vi "Main.vi"() -> ()   [LabVIEW 2014]
uses:
  experimental data.ctl
  <vilib>/Utility/sysdir.llb/System Directory Type.ctl
  <vilib>/Utility/error.llb/DialogType.ctl
  <vilib>/DAQmx/create/channels.llb/DAQmx Create Channel (AI-Voltage-Basic).vi
  <vilib>/DAQmx/create/channels.llb/DAQmx Create Channel (AO-Voltage-Basic).vi
  <vilib>/DAQmx/configure/timing.llb/DAQmx Timing (Sample Clock).vi
  <vilib>/DAQmx/write.llb/DAQmx Write (Analog DBL 1Chan 1Samp).vi
  <vilib>/Utility/config.llb/NI_LVConfig.lvlib
panel:
  out "Progress":string
  in  "Send email":bool
  in  "Email recipient":string
  in  "Number of loops to average":u16=8 min=1 step=1
  in  "Scan comments":string="These comments are saved on the screenshot image, and get emailed to you, but are NOT saved to the text data file. You have been warned."
  out "Last scan saved as":path=path "C:/Users/rajv202/Downloads/MOKE Data/2014-12-04/164027.dat"
  out "A-B Graph":cluster{dbl[], dbl[]}(graph)={[-0.07477034821619312, -0.04425183874019593, -0.013733329264198737, 0.016479995117038484, 0.04699850459303567, 0.07751701406903287, 0.10788293099765008, 0.13840144047364727, 0.16876735740226448, 0.19928586687826166, 0.22965178380687887, 0.26001770073549607, 0.2903836176641133, 0.32090212714011046, 0.3511154515213477, 0.3814813684499649, 0.4118472853785821, 0.4422132023071993, 0.47242652668843654, 0.5027924436170538, 0.5330057679982909, 0.5632190923795282, 0.5934324167607654, 0.6234931485946227, 0.6537064729758598, 0.6837672048097171, 0.7138279366435744, 0.7438886684774315, 0.7739494003112888, 0.804010132145146, 0.8339182714316232, 0.8638264107181005, 0.8937345500045778, 0.923490096743675, 0.9533982360301523, 0.9831537827692496, 1.012756736960967, 1.042512283700064, 1.0721152378917813, 1.1017181920834986, 1.131321146275216, 1.1607715079195533, 1.1902218695638904, 1.2195196386608478, 1.2489700003051851, 1.2782677694021425, 1.3074129459517196, 1.336710715048677, 1.3657032990508744, 1.3948484756004518, 1.423841059602649, 1.4528336436048463, 1.4816736350596638, 1.510513626514481, 1.5393536179692984, 1.5680410168767358, 1.596575823236793, 1.6252632221442305, 1.653645435956908, 1.6821802423169652, 1.7105624561296426, 1.7387920773949401, 1.7670216986602374, 1.7952513199255349, 1.8233283486434522, 1.8512527848139897, 1.8791772209845272, 1.9071016571550645, 1.934873500778222, 1.9624927518539994, 1.990112002929777, 2.0177312540055543, 2.045197912533952, 2.0725119785149695, 2.0998260444959866, 2.1269875179296243, 2.154148991363262, 2.1811578722495195, 2.2080141605883967, 2.2348704489272744, 2.261574144718772, 2.2882778405102693, 2.314828943754387, 2.3413800469985047, 2.3676259651478624, 2.3940244758445997, 2.4201178014465774, 2.446211127048555, 2.4721518601031525, 2.4980925931577502, 2.523880733664968, 2.5495162816248054, 2.575151829584643, 2.6006347849971005, 2.6259651478621784, 2.6511429181798762, 2.6763206884975737, 2.7013458662678915, 2.726371044038209, 2.751091036713767, 2.775811029389325, 2.8005310220648822, 2.82494582964568, 2.8493606372264777, 2.8736228522598957, 2.897732474745933, 2.921689504684591, 2.945646534623249, 2.969450972014527, 2.993102816858425, 3.0166020691549424, 3.0401013214514605, 3.063295388653218, 3.0864894558549762, 3.109530930509354, 3.1324198126163516, 3.1553086947233497, 3.1778923917355875, 3.2004760887478256, 3.2229071932126834, 3.2451857051301616, 3.2673116245002594, 3.2892849513229776, 3.3112582781456954, 3.3329264198736532, 3.3545945616016115, 3.3761101107821894, 3.3974730674153872, 3.4186834315012056, 3.4397412030396435, 3.4606463820307014, 3.48139896847438, 3.5019989623706778, 3.5225989562669757, 3.542893765068514, 3.563188573870052, 3.58317819757683, 3.6031678212836087, 3.6230048524430067, 3.642536698507645, 3.662068544572283, 3.6814477980895415, 3.7006744590594196, 3.7197485274819178, 3.738670003357036, 3.757438886684774, 3.7759025849177528, 3.794366283150731, 3.8126773888363292, 3.8308359019745475, 3.8488418225653858, 3.866695150608844, 3.884395886104923, 3.901944029053621, 3.9191869869075595, 3.936429944761498, 3.9535203100680563, 3.9704580828272347, 3.987090670491653, 4.0037232581560716, 4.0200506607257305, 4.0363780632953885, 4.0524002807702875, 4.0684224982451855, 4.0841395306253245, 4.099703970458083, 4.115115817743462, 4.13037507248146, 4.145481734672079, 4.160435804315317, 4.175237281411176, 4.1897335734122745, 4.204229865413374, 4.218420972319712, 4.23261207922605, 4.246498001037629], [0.7960753196813868, 0.8261360515152439, 0.8560441908017212, 0.8859523300881985, 0.9158604693746757, 0.945768608661153, 0.9755241554002503, 1.0052797021393476, 1.0350352488784447, 1.064790795617542, 1.0943937498092593, 1.1239967040009766, 1.153447065645314, 1.183050019837031, 1.2125003814813684, 1.2417981505783258, 1.271248512222663, 1.3005462813196202, 1.3298440504165776, 1.358989226966155, 1.3881344035157324, 1.4171269875179295, 1.446272164067507, 1.4751121555223243, 1.5041047395245217, 1.532944730979339, 1.5616321298867764, 1.5904721213415938, 1.619006927701651, 1.6476943266090884, 1.6762291329691459, 1.7046113467818231, 1.7329935605945006, 1.7613757744071779, 1.7896053956724753, 1.8176824243903928, 1.8459120456556901, 1.8738364818262276, 1.901760917996765, 1.9296853541673025, 1.95745719779046, 1.9852290414136173, 2.012848292489395, 2.0403149510177925, 2.0677816095461896, 2.095248268074587, 2.122562334055605, 2.1497238074892424, 2.1768852809228796, 2.203894161809137, 2.230903042695395, 2.257759331034272, 2.2844630268257697, 2.3111667226172674, 2.337717825861385, 2.3642689291055023, 2.39066743980224, 2.416913357951598, 2.443159276100955, 2.469252601702933, 2.4951933347575306, 2.521134067812128, 2.5469222083193457, 2.5727103488265635, 2.598193304239021, 2.6236762596514787, 2.6491592150639365, 2.674489577929014, 2.6996673482467117, 2.724692526017029, 2.749565111239967, 2.774437696462905, 2.7991576891384624, 2.8238776818140203, 2.848292489394818, 2.8727072969756158, 2.8969695120090333, 2.9212317270424513, 2.945188756981109, 2.969145786919767, 2.992950224311045, 3.0166020691549424, 3.0402539139988405, 3.063600573747978, 3.086947233497116, 3.110141300698874, 3.133182775353252, 3.1562242500076296, 3.1789605395672473, 3.2016968291268655, 3.224280526139103, 3.2467116306039614, 3.268990142521439, 3.2912686544389174, 3.313241981261635, 3.335215308084353, 3.3568834498123112, 3.378551591540269, 3.4000671407208474, 3.4214300973540452, 3.442793053987243, 3.4638508255256815, 3.4847560045167394, 3.5056611835077973, 3.5262611774040957, 3.5468611713003937, 3.5671559801019317, 3.58745078890347, 3.607593005157628, 3.627582628864406, 3.6474196600238042, 3.6671040986358228, 3.686635944700461, 3.706015198217719, 3.725241859187597, 3.7443159276100957, 3.763237403485214, 3.782006286812952, 3.8006225775933102, 3.8190862758262885, 3.837397381511887, 3.8557084871974854, 3.8737144077883237, 3.891567735831782, 3.9092684713278603, 3.9268166142765586, 3.944212164677877, 3.9614551225318158, 3.978545487838374, 3.9954832605975525, 4.0122684408093505, 4.028901028473769, 4.045228431043427, 4.061555833613086, 4.077730643635364, 4.093600268562883, 4.1094698934904015, 4.1250343333231605, 4.140598773155919, 4.155858027893918, 4.170964690084536, 4.185918759727775, 4.200720236823633, 4.215369121372112, 4.2298654133732105, 4.24420911282693, 4.258247627185888, 4.272286141544847, 4.2860194708090456, 4.299600207525865, 4.313028351695303, 4.326303903317362, 4.339426862392041, 4.352397228919339, 4.365062410351879, 4.377727591784417, 4.390087588122196, 4.402294991912595, 4.414349803155614, 4.426252021851253, 4.438001647999512, 4.44944608905301, 4.46089053010651, 4.4720297860652485, 4.483016449476607, 4.493850520340587, 4.5043794061098055, 4.514908291879024, 4.525131992553484, 4.535203100680563, 4.5451216162602615, 4.554887539292581, 4.56450086977752, 4.573809015167699, 4.582964568010499, 4.591967528305918]}
  out "A+B Graph":cluster{dbl[], dbl[]}(graph)={[-0.07477034821619312, -0.04425183874019593, -0.013733329264198737, 0.016479995117038484, 0.04699850459303567, 0.07751701406903287, 0.10788293099765008, 0.13840144047364727, 0.16876735740226448, 0.19928586687826166, 0.22965178380687887, 0.26001770073549607, 0.2903836176641133, 0.32090212714011046, 0.3511154515213477, 0.3814813684499649, 0.4118472853785821, 0.4422132023071993, 0.47242652668843654, 0.5027924436170538, 0.5330057679982909, 0.5632190923795282, 0.5934324167607654, 0.6234931485946227, 0.6537064729758598, 0.6837672048097171, 0.7138279366435744, 0.7438886684774315, 0.7739494003112888, 0.804010132145146, 0.8339182714316232, 0.8638264107181005, 0.8937345500045778, 0.923490096743675, 0.9533982360301523, 0.9831537827692496, 1.012756736960967, 1.042512283700064, 1.0721152378917813, 1.1017181920834986, 1.131321146275216, 1.1607715079195533, 1.1902218695638904, 1.2195196386608478, 1.2489700003051851, 1.2782677694021425, 1.3074129459517196, 1.336710715048677, 1.3657032990508744, 1.3948484756004518, 1.423841059602649, 1.4528336436048463, 1.4816736350596638, 1.510513626514481, 1.5393536179692984, 1.5680410168767358, 1.596575823236793, 1.6252632221442305, 1.653645435956908, 1.6821802423169652, 1.7105624561296426, 1.7387920773949401, 1.7670216986602374, 1.7952513199255349, 1.8233283486434522, 1.8512527848139897, 1.8791772209845272, 1.9071016571550645, 1.934873500778222, 1.9624927518539994, 1.990112002929777, 2.0177312540055543, 2.045197912533952, 2.0725119785149695, 2.0998260444959866, 2.1269875179296243, 2.154148991363262, 2.1811578722495195, 2.2080141605883967, 2.2348704489272744, 2.261574144718772, 2.2882778405102693, 2.314828943754387, 2.3413800469985047, 2.3676259651478624, 2.3940244758445997, 2.4201178014465774, 2.446211127048555, 2.4721518601031525, 2.4980925931577502, 2.523880733664968, 2.5495162816248054, 2.575151829584643, 2.6006347849971005, 2.6259651478621784, 2.6511429181798762, 2.6763206884975737, 2.7013458662678915, 2.726371044038209, 2.751091036713767, 2.775811029389325, 2.8005310220648822, 2.82494582964568, 2.8493606372264777, 2.8736228522598957, 2.897732474745933, 2.921689504684591, 2.945646534623249, 2.969450972014527, 2.993102816858425, 3.0166020691549424, 3.0401013214514605, 3.063295388653218, 3.0864894558549762, 3.109530930509354, 3.1324198126163516, 3.1553086947233497, 3.1778923917355875, 3.2004760887478256, 3.2229071932126834, 3.2451857051301616, 3.2673116245002594, 3.2892849513229776, 3.3112582781456954, 3.3329264198736532, 3.3545945616016115, 3.3761101107821894, 3.3974730674153872, 3.4186834315012056, 3.4397412030396435, 3.4606463820307014, 3.48139896847438, 3.5019989623706778, 3.5225989562669757, 3.542893765068514, 3.563188573870052, 3.58317819757683, 3.6031678212836087, 3.6230048524430067, 3.642536698507645, 3.662068544572283, 3.6814477980895415, 3.7006744590594196, 3.7197485274819178, 3.738670003357036, 3.757438886684774, 3.7759025849177528, 3.794366283150731, 3.8126773888363292, 3.8308359019745475, 3.8488418225653858, 3.866695150608844, 3.884395886104923, 3.901944029053621, 3.9191869869075595, 3.936429944761498, 3.9535203100680563, 3.9704580828272347, 3.987090670491653, 4.0037232581560716, 4.0200506607257305, 4.0363780632953885, 4.0524002807702875, 4.0684224982451855, 4.0841395306253245, 4.099703970458083, 4.115115817743462, 4.13037507248146, 4.145481734672079, 4.160435804315317, 4.175237281411176, 4.1897335734122745, 4.204229865413374, 4.218420972319712, 4.23261207922605, 4.246498001037629], [0.43214209418012023, 0.46250801110873746, 0.49287392803735464, 0.5230872524185919, 0.5534531693472091, 0.5836664937284463, 0.6140324106570635, 0.6442457350383007, 0.674459059419538, 0.7045197912533951, 0.7347331156346324, 0.7647938474684897, 0.7948545793023468, 0.8249153111362041, 0.8549760429700614, 0.8850367748039186, 0.9149449140903958, 0.9448530533768731, 0.9747611926633504, 1.0045167394024477, 1.0344248786889247, 1.064180425428022, 1.0939359721671194, 1.1235389263588367, 1.153141880550554, 1.182744834742271, 1.2123477889339884, 1.2417981505783258, 1.271248512222663, 1.3006988738670002, 1.3299966429639576, 1.359294412060915, 1.3885921811578723, 1.4177373577074495, 1.4468825342570268, 1.4760277108066042, 1.5050202948088016, 1.5338602862636188, 1.5628528702658162, 1.5916928617206336, 1.6203802606280708, 1.6492202520828882, 1.6777550584429457, 1.706442457350383, 1.7348246711630604, 1.7633594775231178, 1.791741691335795, 1.8199713126010926, 1.84820093386639, 1.8764305551316873, 1.9045075838496048, 1.9325846125675221, 1.9605090487380596, 1.988280892361217, 2.0160527359843745, 2.043824579607532, 2.0714438306833096, 2.0989104892117068, 2.1263771477401043, 2.153843806268502, 2.1811578722495195, 2.2083193456831567, 2.2354808191167943, 2.262489700003052, 2.2893459883419296, 2.316202276680807, 2.3430585650196845, 2.369609668263802, 2.3963133640552994, 2.422711874752037, 2.449110385448775, 2.475356303598132, 2.50160222174749, 2.5276955473494676, 2.553636280404065, 2.5795770134586626, 2.6053651539658804, 2.6310007019257178, 2.6566362498855556, 2.6821192052980134, 2.707449568163091, 2.7327799310281686, 2.7579577013458665, 2.782982879116184, 2.807855464339122, 2.8327280495620593, 2.857448042237617, 2.8820154423657947, 2.9065828424939726, 2.9309976500747705, 2.955259865108188, 2.979369487594226, 3.0034791100802636, 3.0272835474715416, 3.051087984862819, 3.074739829706717, 3.098391674550615, 3.121738334299753, 3.1450849940488905, 3.1682790612506486, 3.1913205359050263, 3.2142094180120244, 3.237098300119022, 3.2598345896786403, 3.282265694143498, 3.3046967986083557, 3.326975310525834, 3.3492538224433117, 3.37122714926603, 3.3932004760887478, 3.414868617816706, 3.436536759544664, 3.4580523087252417, 3.47941526535844, 3.500625629444258, 3.521683400982696, 3.542588579973754, 3.563493758964812, 3.58409375286111, 3.6046937467574085, 3.6249885555589465, 3.6452833643604845, 3.665425580614643, 3.685262611774041, 3.705099642933439, 3.724784081545457, 3.7443159276100957, 3.763695181127354, 3.782921842097232, 3.80199591051973, 3.8209173863948487, 3.839686269722587, 3.858302560502945, 3.8767662587359233, 3.8950773644215215, 3.91323587755974, 3.9312417981505785, 3.949095126194037, 3.966795861690115, 3.9843440046388134, 4.001739555040132, 4.018829920346691, 4.035920285653249, 4.052858058412427, 4.069643238624225, 4.086275826288644, 4.102603228858302, 4.118930631427961, 4.134952848902859, 4.150975066377758, 4.166692098757896, 4.182409131138035, 4.1978209784234135, 4.213080233161413, 4.228186895352031, 4.24314096499527, 4.257942442091128, 4.272591326639607, 4.286935026093325, 4.301278725547045, 4.315317239906003, 4.329355754264962, 4.3430890835291605, 4.356669820245979, 4.370097964415418, 4.3833735160374765, 4.396496475112156, 4.409314249092074, 4.422132023071994, 4.434644611957152, 4.447004608294931, 4.45921201208533, 4.471266823328349, 4.483169042023987, 4.494766075624867, 4.506363109225745]}
  out "Estimated finish time":timestamp=timestamp(3500556027.964023 s since 1904-01-01) format="%<%I:%M %p>T"
  out "Progress Bar":u8(slide)=100 scale=0.0..100.0
  in  "Stop Button":bool
  in  "Magnet Ramp Segments":string[][](table)=[["0", "-1", "8"], ["-1", "1", "80"], ["1", "-1", "80"], ["-1", "0", "8"]]
  in  "Field Settle Time (msec)":dbl=400.0
  in  "Output Voltage Limit +/-":dbl=5.0 min=0.0 max=10.0 step=0.0001 format="%.2f"
  in  "Input Voltage Limit +/-":dbl=5.0 min=0.0 max=10.0 step=0.0001 format="%.2f"
  in  "Magnet Power Supply Channel":tag="Dev1/ao0"
  in  "A-B Channel":tag="Dev1/ai1"
  in  "A+B Channel":tag="Dev1/ai0"
  in  "Hall Probe Channel":tag="Dev1/ai2"
  in  "Start Button":bool
  # "Generic Small MOKE"
  # "Released 2015-01-16 16:23"
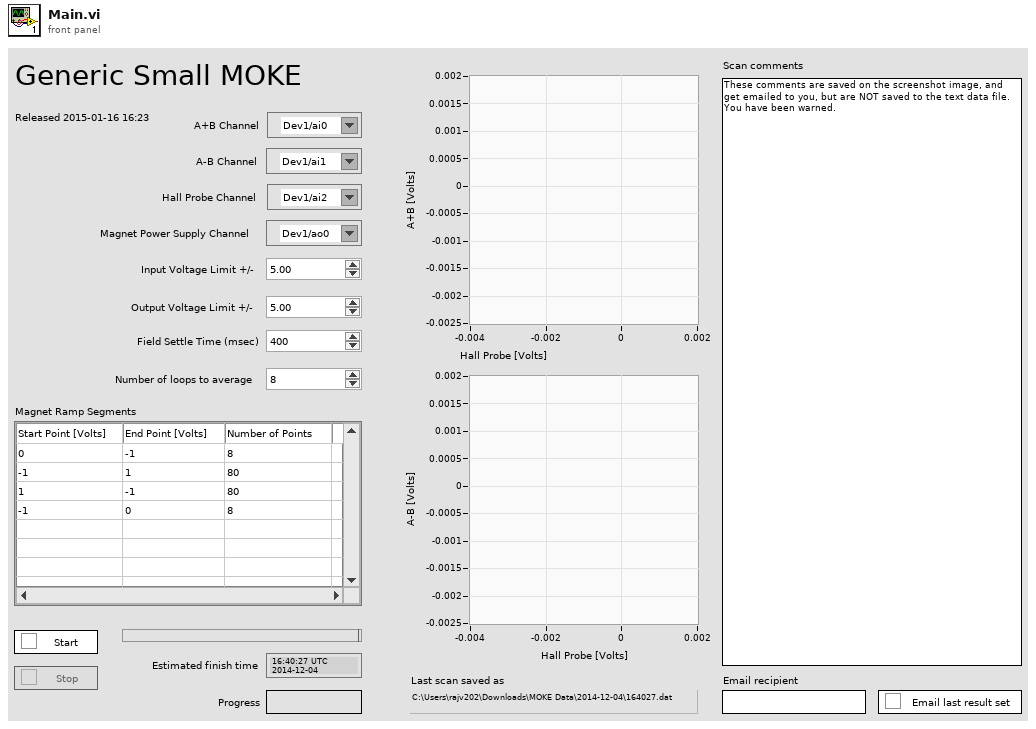
[diagram p1: front panel]
types:
  T1 = typedef "System Directory Type.ctl" = i32
  T2 = typedef "experimental data.ctl" = cluster{"Hall Probe":dbl, "A+B":dbl, "A-B":dbl, "Progress":u32[]}
  T3 = typedef "NI_LVConfig.lvlib/Config Data RefNum.ctl" = refnum<k1>
  T4 = enum8{"Enabled", "Disabled", "Disabled and Grayed Out"}
  T5 = enum16{"open", "replace", "create", "open or create", "replace or create", "replace or create with confirmation"}
  T6 = typedef "imagedata.ctl" = cluster{"image type":i32, "image depth":i32, "image":u8[], "mask":u8[], "colors":u32[], "Rectangle":cluster{"left":i16, "top":i16, "right":i16, "bottom":i16}}
  T7 = typedef "DialogType.ctl" = u16
  T8 = cluster{"New data array":dbl[], "New data array":dbl[]}
  T9 = cluster{"Server address":string, "Use TLS?":bool, "Username":string, "Password":string, "Recipient":string}
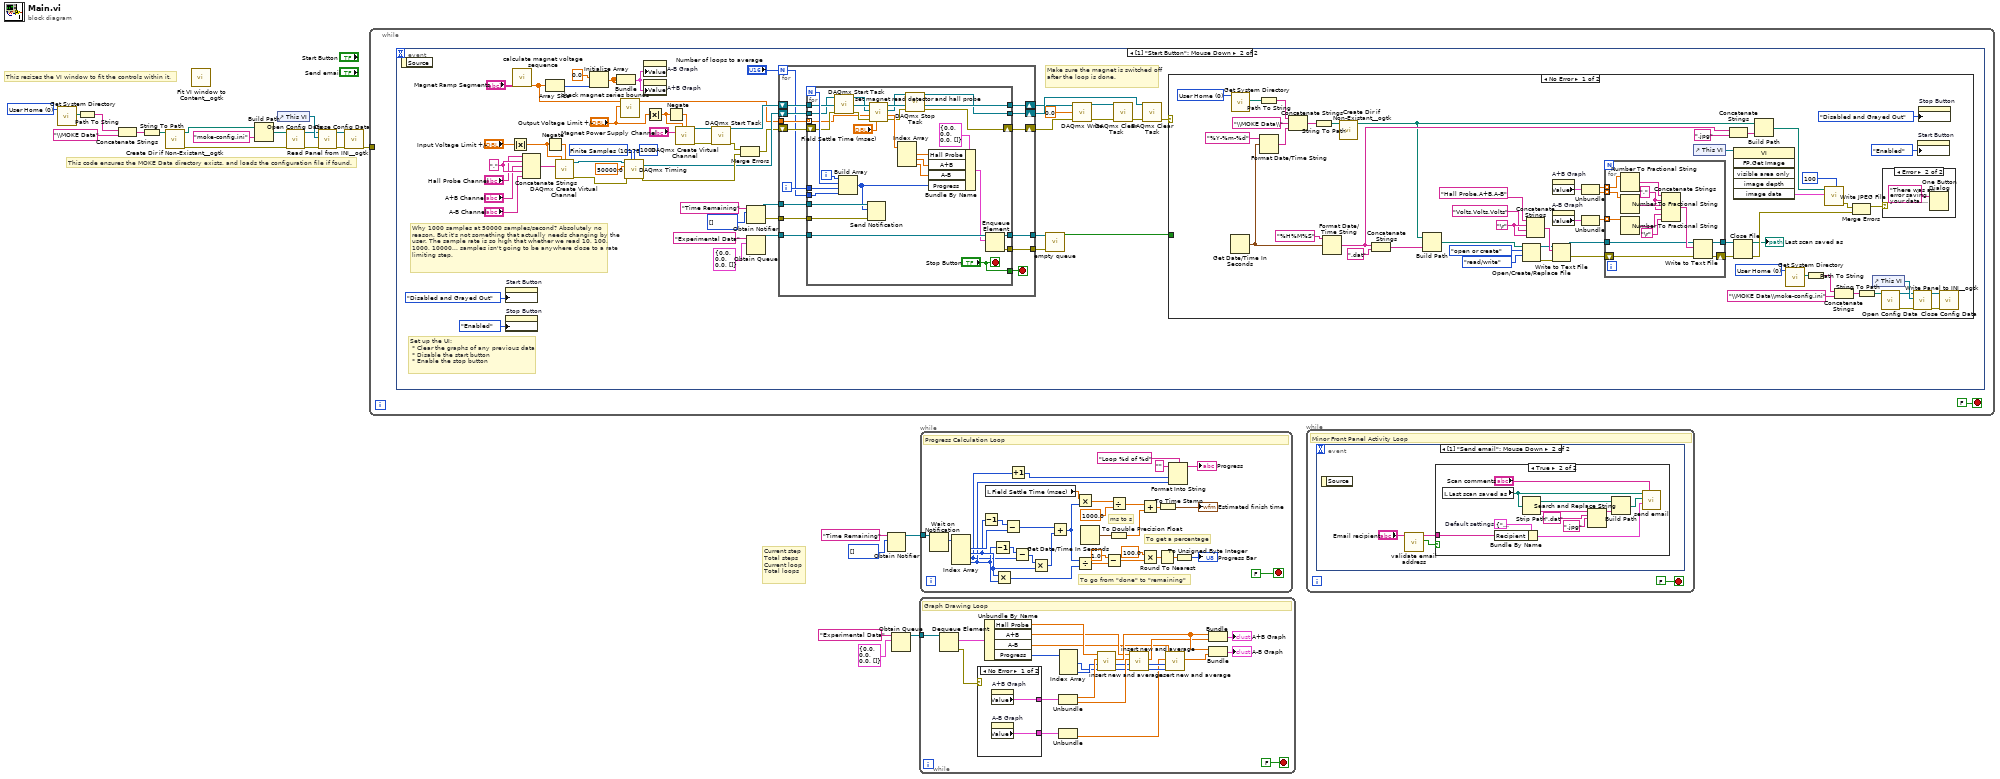
[diagram p0: block diagram]
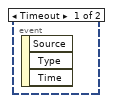
[diagram p2: hidden frame]
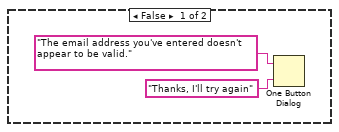
[diagram p3: hidden frame]
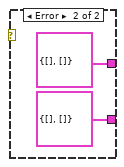
[diagram p4: hidden frame]
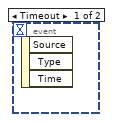
[diagram p5: hidden frame]
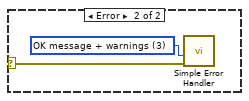
[diagram p7: hidden frame]
diagram:
  w16 = T1 0 items=["User Home"=0, "User Desktop"=1, "User Documents"=2, "User Application Data"=3, "User Preferences"=4, "User Temporary"=5, "Public Documents"=6, "Public Application Data"=7, "Public Preferences"=8, "Public Cache"=13, "System Core Libraries"=9, "System Installed Libraries"=10, "Application Files"=11, "Boot Volume Root"=12] ("system directory type")
  # "This code ensures the MOKE Data directory exists, and loads the configuration file if found."
  # "This resizes the VI window to fit the controls within it."
  # "Current step\nTotal steps\nCurrent loop\nTotal loops"
  n1 = call <vilib>:"Get System Directory.vi"("system directory type"=w16) -> ("system directory"=w15:path)  [unwired: 10 in]
  n2 = Path To String(path=w15) -> (string=w14:string)
  n3 = Concatenate Strings(w14, "\\MOKE Data" ("string")) -> (w13:string)
  n4 = String To Path(string=w13) -> (path=w5:path)
  n5 = call <userlib>:"Create Dir if Non-Existant__ogtk.vi"("Directory Path"=w5) -> ("error out"=w4:errorcluster, "dup Directory Path"=w2:path)  [unwired: 8 in, 1 out]
  n6 = call <userlib>:"Fit VI window to Content__ogtk.vi"() -> ()  [unwired: 6 in, 2 out]
  n7 = Build Path(base path=w2, name or relative path="moke-config.ini") -> (appended path=w3:path)
  n8 = control-ref of="This VI"() -> (w12:refnum<vi>)
  n9 = call <vilib>:"Open Config Data.vi"("error in (no error)"=w4, "configuration file path"=w3) -> ("error out"=w10:errorcluster, "refnum"=w11:T3)  [unwired: 7 in, 1 out]
  n10 = call <userlib>:"Read Panel from INI__ogtk.vi"("error in (no error)"=w10, "VI ref"=w12, "refnum"=w11) -> ("error out"=w8:errorcluster, "refnum out"=w9:T3)  [unwired: 7 in]
  n11 = call <vilib>:"Close Config Data.vi"("error in (no error)"=w8, "refnum"=w9) -> ("error out"=w6:errorcluster)  [unwired: 8 in, 1 out]
  n12 = while {
    tunnel: w6 -> [_]
    stop <- FALSE stop-if-true
    n13 = event shown="[1] \"Start Button\": Mouse Down" {
      selector: _ -> [_ _]
      dyn-events: _ -> [_ _]
      timeout: _ -> [_ _]
      event Timeout {
        n14 = event-data() -> ()  [unwired: 1 in, 3 out]
      }
      event "Start Button": Mouse Down {
        w34 = 10178 items=["Finite Samples"=10178, "Continuous Samples"=10123, "Hardware Timed Single Point"=12522] ("sample mode")
        w75 = ","
        # "Why 1000 samples at 50000 samples/second? Absolutely no reason. But it's not something that actually needs changing by the user. The sample rate is so high that whether we read 10, 100, 1000, 10000... samples isn't going to be anywhere close to a rate limiting step."
        # "Make sure the magnet is switched off after the loop is done."
        # "Set up the UI:\n * Clear the graphs of any previous data\n * Disable the start button\n * Enable the stop button"
        n15 = event-data() -> ()  [unwired: 1 in, 1 out]
        n16 = property on="Start Button" class="Bool (strict)"("DisabledEnum"=T4."Disabled and Grayed Out" ("Disabled")) -> ()  [unwired: 2 in, 2 out]
        n17 = property on="Stop Button" class="Bool"("DisabledEnum"=T4."Enabled" ("Disabled")) -> ()  [unwired: 2 in, 2 out]
        n18 = Absolute Value(x="Input Voltage Limit +/-") -> (abs(x)=w68:dbl)
        n19 = call "calculate magnet voltage sequence.vi"("Magnet Ramp Segments"="Magnet Ramp Segments") -> ("Magnet Voltage Sequence"=w36:dbl[])  [unwired: 8 in]
        n20 = Concatenate Strings("Hall Probe Channel", w75, "A+B Channel", w75, "A-B Channel") -> (w71:string)
        n21 = Array Size(array=w36) -> (size(s)=w42:i32)
        n22 = Negate(x=w68) -> (-x=w70:dbl)
        n23 = call-poly <vilib>:"DAQmx Create Virtual Channel.vi"("maximum value"=w68, "minimum value"=w70, "physical channels"=w71) -> ("task out"=w35:refnum<k21>, "error out"=w32:errorcluster)  [unwired: 11 in]
        n24 = Initialize Array(0.0 ("element"), w42) -> (w41:dbl[])
        n25 = Bundle(w41, w41) -> (w40:cluster{dbl[], dbl[]})  [unwired: 1 in]
        n26 = call "check magnet series bounds.vi"("Output Voltage Limit"="Output Voltage Limit +/-", "Magnet Voltage Sequence"=w36) -> ("Magnet Voltage Sequence"=w27:dbl[])  [unwired: 9 in]
        n27 = call-poly <vilib>:"DAQmx Timing.vi"("task/channels in"=w35, "sample mode"=w34, "samples per channel"=1000, "rate"=50000.0, "error in"=w32) -> ("task out"=w30:refnum<k21>, "error out"=w31:errorcluster)  [unwired: 9 in]
        n28 = property on="A-B Graph" class="XYGraph (strict)"("Value"=w40) -> ()  [unwired: 2 in, 2 out]
        n29 = property on="A+B Graph" class="XYGraph (strict)"("Value"=w40) -> ()  [unwired: 2 in, 2 out]
        n30 = Absolute Value(x="Output Voltage Limit +/-") -> (abs(x)=w66:dbl)
        n31 = Negate(x=w66) -> (-x=w67:dbl)
        n32 = call-poly <vilib>:"DAQmx Create Virtual Channel.vi"("maximum value"=w66, "minimum value"=w67, "physical channels"="Magnet Power Supply Channel") -> ("task out"=w52:refnum<k21>, "error out"=w65:errorcluster)  [unwired: 11 in]
        n33 = call <vilib>:"DAQmx Start Task.vi"("task/channels in"=w52, "error in"=w65) -> ("task out"=w63:refnum<k21>, "error out"=w64:errorcluster)  [unwired: 12 in]
        n34 = Merge Errors(w64, w31) -> (w29:errorcluster)
        n35 = Obtain Notifier(name (unnamed)="Time Remaining", notification data type=i32[] []) -> (notifier out=w59:refnum<notifier>, error out=w46:errorcluster)  [unwired: 2 in, 1 out]
        n36 = Obtain Queue(name (unnamed)="Experimental Data", element data type=T2 {"Hall Probe"=0.0, "A+B"=0.0, "A-B"=0.0, "Progress"=[]}) -> (queue out=w55:refnum<queue>)  [unwired: 3 in, 2 out]
        n37 = for {
          N: "Number of loops to average" -> [w78]
          tunnel: w59 -> [w87]
          tunnel: w27 -> [w86]
          tunnel: w55 -> [w85]
          tunnel: w46 -> [w81]
          shift-right: [w84] -> w54
          shift-left: w30 -> [w90]
          shift-right: [w82] -> w48
          shift-left: w63 -> [w89]
          shift-right: [w83] -> w51
          shift-left: w29 -> [w88]
          tunnel: [w77] -> w39
          tunnel: [w76] -> w38
          i -> [w79]
          stop <- w80 stop-if-true
          n38 = for {
            N -> [w117]
            tunnel: w90 -> [w95]
            tunnel: w89 -> [w115]
            shift-right: [w99] -> w83
            shift-left: w88 -> [w93]
            tunnel: w86 -> [w91] mode=indexing
            tunnel: w87 -> [w119]
            tunnel: w85 -> [w116]
            tunnel: [w114] -> w82
            tunnel: [w96] -> w84
            tunnel: w81 -> [w112]
            tunnel: ["Stop Button"] -> w80
            tunnel: w79 -> [w108]
            tunnel: w78 -> [w107]
            tunnel: [w103] -> w77
            tunnel: [w102] -> w76
            i -> [w118]
            stop <- "Stop Button" stop-if-true
            n39 = call <vilib>:"DAQmx Start Task.vi"("task/channels in"=w95, "error in"=w93) -> ("task out"=w94:refnum<k21>, "error out"=w92:errorcluster)  [unwired: 12 in]
            n40 = Build Array(w118, w117, w108, w107) -> (w104:i32[])
            n41 = Send Notification(notification=w104, notifier=w119, error in (no error)=w112) -> ()  [unwired: 2 out]
            n42 = call "set magnet read detector and hall probe.vi"("Field settle time (400 msec)"="Field Settle Time (msec)", "error in (no error)"=w92, "Magnet voltage"=w91, "Input task"=w94, "Output task"=w115) -> ("error out"=w98:errorcluster, "Data"=w111:dbl[], "Input task"=w97:refnum<k21>, "Output task"=w114:refnum<k21>)  [unwired: 3 in]
            n43 = Index Array(array=w111) -> (element #1=w106:dbl, element #2=w100:dbl, element #3=w105:dbl)  [unwired: 3 in]
            n44 = call <vilib>:"DAQmx Stop Task.vi"("task/channels in"=w97, "error in"=w98) -> ("task out"=w96:refnum<k21>, "error out"=w99:errorcluster)  [unwired: 12 in]
            n45 = Bundle By Name(cluster=T2 {"Hall Probe"=0.0, "A+B"=0.0, "A-B"=0.0, "Progress"=[]}, "Hall Probe"=w106, "A+B"=w100, "A-B"=w105, "Progress"=w104) -> (w109:T2)
            n46 = Enqueue Element(queue=w116, element=w109) -> (queue out=w102:refnum<queue>, error out=w103:errorcluster)  [unwired: 2 in, 1 out]
          }
        }
        n47 = call "empty queue.vi"("error in (no error)"=w39, "Queue in"=w38) -> ("Queue emptied?"=w37:bool)  [unwired: 9 in]
        n48 = call-poly <vilib>:"DAQmx Write.vi"("task/channels in"=w48, "data"=0.0, "error in"=w51) -> ("task out"=w49:refnum<k21>, "error out"=w50:errorcluster)  [unwired: 10 in, 1 out]
        n49 = call <vilib>:"DAQmx Clear Task.vi"("task in"=w49, "error in"=w50) -> ("error out"=w62:errorcluster)  [unwired: 13 in]
        n50 = call <vilib>:"DAQmx Clear Task.vi"("task in"=w54, "error in"=w62) -> ("error out"=w24:errorcluster)  [unwired: 13 in]
        n51 = case shown="No Error" w24 {
          selector: w24 -> [_ w189]
          tunnel: w37 -> [_ _]
          frame No Error {
            w138 = T1 0 items=["User Home"=0, "User Desktop"=1, "User Documents"=2, "User Application Data"=3, "User Preferences"=4, "User Temporary"=5, "Public Documents"=6, "Public Application Data"=7, "Public Preferences"=8, "Public Cache"=13, "System Core Libraries"=9, "System Installed Libraries"=10, "Application Files"=11, "Boot Volume Root"=12] ("system directory type")
            w141 = T1 0 items=["User Home"=0, "User Desktop"=1, "User Documents"=2, "User Application Data"=3, "User Preferences"=4, "User Temporary"=5, "Public Documents"=6, "Public Application Data"=7, "Public Preferences"=8, "Public Cache"=13, "System Core Libraries"=9, "System Installed Libraries"=10, "Application Files"=11, "Boot Volume Root"=12] ("system directory type")
            w147 = "\r"
            n52 = Get Date/Time In Seconds() -> (seconds since 1Jan1904=w172:timestamp)
            n53 = call <vilib>:"Get System Directory.vi"("system directory type"=w141) -> ("system directory"=w140:path)  [unwired: 10 in]
            n54 = Path To String(path=w140) -> (string=w139:string)
            n55 = Format Date/Time String(time format string (%c)="%Y-%m-%d", seconds (now)=w172) -> (date/time string=w124:string)  [unwired: 1 in]
            n56 = Concatenate Strings(w139, "\\MOKE Data\\" ("string"), w124) -> (w134:string)
            n57 = String To Path(string=w134) -> (path=w173:path)
            n58 = Format Date/Time String(time format string (%c)="%H%M%S", seconds (now)=w172) -> (date/time string=w153:string)  [unwired: 1 in]
            n59 = call <userlib>:"Create Dir if Non-Existant__ogtk.vi"("Directory Path"=w173) -> ("dup Directory Path"=w151:path)  [unwired: 8 in, 2 out]
            n60 = Concatenate Strings(w153, ".dat" ("string")) -> (w170:string)
            n61 = Build Path(base path=w151, name or relative path=w170) -> (appended path=w144:path)
            n62 = Open/Create/Replace File(file path (use dialog)=w144, operation (0:open)=T5."open or create", access (0:read/write)=enum16{"read/write", "read-only", "write-only"}."read/write") -> (refnum out=w164:refnum<file>, error out=w165:errorcluster)  [unwired: 3 in, 1 out]
            n63 = Concatenate Strings("Hall Probe,A+B,A-B" ("text"), w147, "Volts,Volts,Volts" ("string"), w147) -> (w166:string)
            n64 = property on="A+B Graph" class="XYGraph (strict)"() -> ("Value"=w163:cluster{dbl[], dbl[]})  [unwired: 2 in, 2 out]
            n65 = property on="A-B Graph" class="XYGraph (strict)"() -> ("Value"=w162:cluster{dbl[], dbl[]})  [unwired: 2 in, 2 out]
            n66 = Write to Text File(file (use dialog)=w164, text=w166, error in=w165) -> (refnum out=w158:refnum<file>, error out=w123:errorcluster)  [unwired: 1 in, 1 out]
            n67 = Unbundle(w163) -> (w161:dbl[], w160:dbl[])
            n68 = Unbundle(w162) -> (w159:dbl[])  [unwired: 1 out]
            n69 = for {
              tunnel: w161 -> [w188] mode=indexing
              tunnel: w160 -> [w187] mode=indexing
              tunnel: w159 -> [w186] mode=indexing
              tunnel: w158 -> [w179]
              tunnel: [w178] -> w157
              shift-right: [w176] -> w122
              shift-left: w123 -> [w177]
              w182 = "," ("string")
              n70 = Number To Fractional String(number=w188) -> (F-format string=w185:string)  [unwired: 3 in]
              n71 = Number To Fractional String(number=w187) -> (F-format string=w184:string)  [unwired: 3 in]
              n72 = Number To Fractional String(number=w186) -> (F-format string=w183:string)  [unwired: 3 in]
              n73 = Concatenate Strings(w185, w182, w184, w182, w183, "\r") -> (w180:string)
              n74 = Write to Text File(file (use dialog)=w179, text=w180, error in=w177) -> (refnum out=w178:refnum<file>, error out=w176:errorcluster)  [unwired: 1 in, 1 out]
            }
            n75 = control-ref of="This VI"() -> (w155:refnum<vi>)
            n76 = Concatenate Strings(w153, ".jpg" ("string")) -> (w152:string)
            n77 = invoke on="Invoke Node" class="VI" method="FP.Get Image"(reference=w155) -> ("image data"=w156:T6)  [unwired: 5 in, 5 out]
            n78 = Close File(refnum=w157, error in=w122) -> (path=→"Last scan saved as":path, error out=w142:errorcluster)
            n79 = Build Path(base path=w151, name or relative path=w152) -> (appended path=w150:path)
            n80 = call <vilib>:"Get System Directory.vi"("system directory type"=w138) -> ("system directory"=w137:path)  [unwired: 10 in]
            n81 = Path To String(path=w137) -> (string=w136:string)
            n82 = call <vilib>:"Write JPEG File.vi"("quality (80)"=100, "image data"=w156, "path to JPEG file"=w150) -> ("error out"=w143:errorcluster)  [unwired: 7 in, 1 out]
            n83 = Concatenate Strings(w136, "\\MOKE Data\\moke-config.ini" ("string")) -> (w135:string)
            n84 = Merge Errors(w143, w142) -> (w133:errorcluster)
            n85 = String To Path(string=w135) -> (path=w129:path)
            n86 = control-ref of="This VI"() -> (w132:refnum<vi>)
            n87 = call <vilib>:"Open Config Data.vi"("configuration file path"=w129) -> ("error out"=w130:errorcluster, "refnum"=w131:T3)  [unwired: 8 in, 1 out]
            n88 = case shown="Error" w133 {
              frame No Error {
              }
              frame Error {
                n89 = One Button Dialog(message="There was an error saving your data. PLEASE check that the last data file and screenshot saved successfully if the data are important to you.") -> ()  [unwired: 1 in, 1 out]
              }
            }
            n90 = call <userlib>:"Write Panel to INI__ogtk.vi"("error in (no error)"=w130, "VI ref"=w132, "refnum"=w131) -> ("error out"=w127:errorcluster, "refnum out"=w128:T3)  [unwired: 7 in]
            n91 = property on="Start Button" class="Bool (strict)"("DisabledEnum"=T4."Enabled" ("Disabled")) -> ()  [unwired: 2 in, 2 out]
            n92 = property on="Stop Button" class="Bool"("DisabledEnum"=T4."Disabled and Grayed Out" ("Disabled")) -> ()  [unwired: 2 in, 2 out]
            n93 = call <vilib>:"Close Config Data.vi"("error in (no error)"=w127, "refnum"=w128) -> ()  [unwired: 8 in, 2 out]
          }
          frame Error {
            w190 = T7 3 items=["no dialog", "OK message", "continue or stop message", "OK message + warnings", "continue/stop + warnings"] ("type of dialog (OK msg:1)")
            n94 = call <vilib>:"Simple Error Handler.vi"("type of dialog (OK msg:1)"=w190, "error in (no error)"=w189) -> ()  [unwired: 3 in, 5 out]
          }
        }
      }
    }
  }
  n95 = Obtain Notifier(name (unnamed)="Time Remaining", notification data type=i32[] []) -> (notifier out=w21:refnum<notifier>)  [unwired: 2 in, 2 out]
  n96 = Obtain Queue(name (unnamed)="Experimental Data", element data type=T2 {"Hall Probe"=0.0, "A+B"=0.0, "A-B"=0.0, "Progress"=[]}) -> (queue out=w17:refnum<queue>)  [unwired: 3 in, 2 out]
  n97 = while {
    tunnel: w17 -> [w213]
    stop <- FALSE stop-if-true
    # "Graph Drawing Loop"
    n98 = Dequeue Element(queue=w213) -> (element=w209:T2, error out=w210:errorcluster)  [unwired: 2 in, 2 out]
    n99 = case shown="No Error" w210 {
      tunnel: [w216 cluster{dbl[], dbl[]} {[], []} ("A-B Graph")] -> w212
      tunnel: [w215 cluster{dbl[], dbl[]} {[], []} ("A-B Graph")] -> w211
      frame No Error {
        n100 = property on="A+B Graph" class="XYGraph (strict)"() -> ("Value"=w216:cluster{dbl[], dbl[]})  [unwired: 2 in, 2 out]
        n101 = property on="A-B Graph" class="XYGraph (strict)"() -> ("Value"=w215:cluster{dbl[], dbl[]})  [unwired: 2 in, 2 out]
      }
      frame Error {
      }
    }
    n102 = Unbundle By Name(w209) -> ("Hall Probe"=w205:dbl, "A+B"=w200:dbl, "A-B"=w193:dbl, "Progress"=w206:u32[])
    n103 = Unbundle(w212) -> (w204:dbl[], w199:dbl[])
    n104 = Unbundle(w211) -> (w192:dbl[])  [unwired: 1 out]
    n105 = Index Array(array=w206) -> (element #1=w201:u32, element #3=w202:u32)  [unwired: 3 in, 1 out]
    n106 = call "insert new and average.vi"("Current step number"=w201, "Current loop number"=w202, "Current data array"=w204, "Value to insert"=w205) -> ("Current step number"=w196:u32, "Current loop number"=w197:u32, "New data array"=w203:dbl[])  [unwired: 5 in]
    n107 = call "insert new and average.vi"("Current step number"=w196, "Current loop number"=w197, "Current data array"=w199, "Value to insert"=w200) -> ("Current step number"=w194:u32, "Current loop number"=w195:u32, "New data array"=w198:dbl[])  [unwired: 5 in]
    n108 = call "insert new and average.vi"("Current step number"=w194, "Current loop number"=w195, "Current data array"=w192, "Value to insert"=w193) -> ("New data array"=w191:dbl[])  [unwired: 5 in, 2 out]
    n109 = Bundle("New data array"=w203, "New data array"=w198) -> (→"A+B Graph":T8)  [unwired: 1 in]
    n110 = Bundle("New data array"=w203, "New data array"=w191) -> (→"A-B Graph":T8)  [unwired: 1 in]
  }
  n111 = while {
    tunnel: w21 -> [w251]
    stop <- FALSE stop-if-true
    # "To get a percentage"
    # "To go from \"done\" to \"remaining\""
    # "ms to s"
    # "Progress Calculation Loop"
    n112 = Wait on Notification(notifier=w251) -> (notification=w243:i32[])  [unwired: 3 in, 3 out]
    n113 = Index Array(array=w243) -> (element #1=w228:i32, element #2=w227:i32, element #3=w220:i32, element #4=w221:i32)  [unwired: 4 in]
    n114 = Decrement(x=w227) -> (x-1=w229:i32)
    n115 = local read "Field Settle Time (msec)"() -> (w226:dbl)
    n116 = Decrement(x=w221) -> (x-1=w239:i32)
    n117 = Multiply(x=w227, y=w221) -> (x*y=w233:i32)
    n118 = Subtract(x=w229, y=w228) -> (x-y=w234:i32)
    n119 = Increment(x=w220) -> (x+1=w219:i32)
    n120 = Subtract(x=w239, y=w220) -> (x-y=w236:i32)
    n121 = Multiply(x=w236, y=w227) -> (x*y=w235:i32)
    n122 = Add(x=w234, y=w235) -> (x+y=w225:i32)
    n123 = Multiply(x=w226, y=w225) -> (x*y=w238:dbl)
    n124 = Divide(x=w225, y=w233) -> (x/y=w231:dbl)
    n125 = Get Date/Time In Seconds() -> (seconds since 1Jan1904=w242:timestamp)
    n126 = Subtract(x=1.0, y=w231) -> (x-y=w232:dbl)
    n127 = Divide(x=w238, y=1000.0 ("x")) -> (x/y=w249:dbl)
    n128 = To Double Precision Float(number=w242) -> (double precision float=w250:dbl)
    n129 = Add(x=w249, y=w250) -> (x+y=w248:dbl)
    n130 = Multiply(x=100.0, y=w232) -> (x*y=w244:dbl)
    n131 = Round To Nearest(number=w244) -> (nearest integer value=w241:dbl)
    n132 = To Time Stamp(1:w248) -> (0:→"Estimated finish time":timestamp)
    n133 = Format Into String(format string="Loop %d of %d", initial string="", w219, w221) -> (resulting string=→"Progress":string)  [unwired: 1 in, 1 out]
    n134 = To Unsigned Byte Integer(number=w241) -> (unsigned 8bit integer=→"Progress Bar":u8)
  }
  n135 = while {
    stop <- FALSE stop-if-true
    # "Minor Front Panel Activity Loop"
    n136 = event shown="[1] \"Send email\": Mouse Down" {
      selector: _ -> [_ _]
      dyn-events: _ -> [_ _]
      timeout: _ -> [_ _]
      event Timeout {
        n137 = event-data() -> ()  [unwired: 1 in, 3 out]
      }
      event "Send email": Mouse Down {
        n138 = event-data() -> ()  [unwired: 1 in, 1 out]
        n139 = call "validate email address.vi"("Email address in"="Email recipient") -> ("Valid?"=w255:bool, "Email address out"=w254:string)  [unwired: 9 in]
        n140 = case shown="True" w255 {
          tunnel: w254 -> [_ w258]
          frame False {
            n141 = One Button Dialog(message="The email address you've entered doesn't appear to be valid.", button name ("OK")="Thanks, I'll try again") -> ()  [unwired: 1 out]
          }
          frame True {
            w259 = T9 {"Server address"="smtp.gmail.com:587", "Use TLS?"=TRUE, "Username"="g24smallmoke@gmail.com", "Password"="IhateLabVIEW", "Recipient"="g24smallmoke@gmail.com"}  # Default settings
            n142 = local read "Last scan saved as"() -> (w262:path)
            n143 = Bundle By Name(cluster=w259, "Recipient"=w258) -> (w260:T9)
            n144 = Strip Path(path=w262) -> (stripped path=w266:path, name=w263:string)
            n145 = Search and Replace String(input string=w263, search string=".dat", replace string=".jpg" ("replace string (\"\")")) -> (result string=w267:string)  [unwired: 5 in, 3 out]
            n146 = Build Path(base path=w266, name or relative path=w267) -> (appended path=w268:path)
            n147 = call "send email.vi"("Body text"="Scan comments", "Email settings"=w260, "Jpeg"=w268, "Data"=w262) -> ()  [unwired: 7 in, 1 out]
          }
        }
      }
    }
  }
